vi "DiffDriveTrainSim_SetInputs.vi"(8 "BatteryVoltage":dbl=12.0, 9 "Right_Volts":dbl=1.0, 10 "Left_Volts":dbl=1.0, 11 "in DiffDriveTrainSim":T1 {"m_Motor"."Jr_KgM2" format="%13.5p"; "m_Motor"."L_H" format="%13.5p"; "m_Motor"."Kt_NMPerAmp" format="%13.5p"; "m_Motor"."KvINV_RadPerSecPerVolt" format="%13.5p"; "m_Motor"."R_Ohms" format="%13.5p"; "m_Motor"."FreeSpeed_RadPerSec" format="%13.5p"; "m_Motor"."FreeCurrent_Amps" format="%13.5p"; "m_Motor"."StallCurrent_Amps" format="%13.5p"; "m_Motor"."StallTorque_NM" format="%13.5p"; "m_Motor"."nominalVoltage_Volts" format="%13.5p"}) -> (0 "Size Coerced":bool, 3 "out DiffDriveTrainSim":T1 {"m_Motor"."Jr_KgM2" format="%13.5p"; "m_Motor"."L_H" format="%13.5p"; "m_Motor"."Kt_NMPerAmp" format="%13.5p"; "m_Motor"."KvINV_RadPerSecPerVolt" format="%13.5p"; "m_Motor"."R_Ohms" format="%13.5p"; "m_Motor"."FreeSpeed_RadPerSec" format="%13.5p"; "m_Motor"."FreeCurrent_Amps" format="%13.5p"; "m_Motor"."StallCurrent_Amps" format="%13.5p"; "m_Motor"."StallTorque_NM" format="%13.5p"; "m_Motor"."nominalVoltage_Volts" format="%13.5p"})   [LabVIEW 2019, in "Trajectory_Library.lvlib"]
doc: "Sets the applied voltage to the drivetrain. Note that positive voltage must make that side of the drivetrain travel forward (+X).\n \nInputs:\n - DiffDriveTraimSim -- Data cluster\n - leftVoltageVolts -- The left voltage.\n - rightVoltageVolts -- The right voltage.\n - BatteryVoltage -- Current battery voltage (volts) (Default = 12 volts)\n\nOutputs:\n - OutDiffDriveTraimSim -- Updated data cluster.\n - SizeCoerced -- If TRUE, an error occured. Execution may continue."
uses:
  Trajectory_Library.lvlib
  TypeDef/LINEAR_SYSTEM.ctl
  <vilib>/Analysis/Matrix/Datatypes/RealMatrix.ctl
  <vilib>/Analysis/Matrix/NI_Matrix.lvlib
  TypeDef/DCMOTOR.CTL
  TypeDef/DIFF_DRIVE_TRAIN_SIM.ctl
panel:
  # "<States, 1>"
  # "<Outputs, 1>"
  # "<Inputs, 1>"
  # "<Outputs, 1>"
  # "<States,States>"
  # "<States,Inputs>"
  # "<Outputs,States>"
  # "<Outputs,Inputs>"
  # "<States, 1>"
  # "<Outputs, 1>"
  # "<Inputs, 1>"
  # "<Outputs, 1>"
  # "<States,States>"
  # "<States,Inputs>"
  # "<Outputs,States>"
  # "<Outputs,Inputs>"
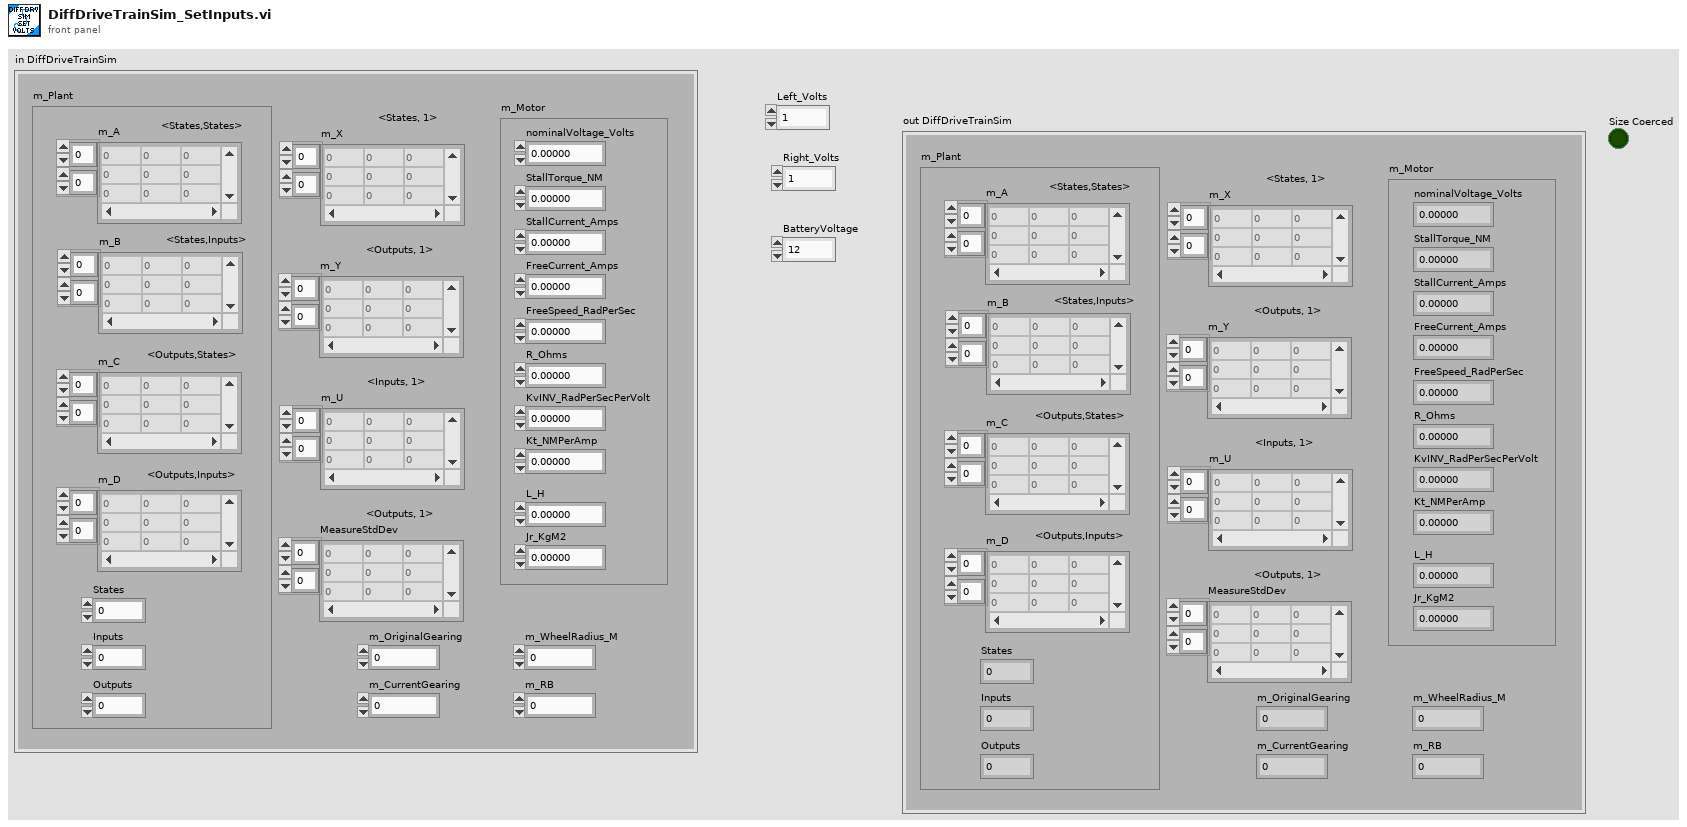
[diagram p1: front panel]
types:
  T1 = typedef "Trajectory_Library.lvlib/DIFF_DRIVE_TRAIN_SIM.ctl" = cluster{"m_Plant":T2, "m_X":T3, "m_Y":T3, "m_U":T3, "MeasureStdDev":T3, "m_Motor":T4, "m_OriginalGearing":dbl, "m_CurrentGearing":dbl, "m_WheelRadius_M":dbl, "m_RB":dbl}
  T2 = typedef "Trajectory_Library.lvlib/LINEAR_SYSTEM.ctl" = cluster{"m_A":T3, "m_B":T3, "m_C":T3, "m_D":T3, "States":i32, "Inputs":i32, "Outputs":i32}
  T3 = typedef "NI_Matrix.lvlib/RealMatrix.ctl" = dbl[][]
  T4 = typedef "Trajectory_Library.lvlib/DCMOTOR.CTL" = cluster{"nominalVoltage_Volts":dbl, "StallTorque_NM":dbl, "StallCurrent_Amps":dbl, "FreeCurrent_Amps":dbl, "FreeSpeed_RadPerSec":dbl, "R_Ohms":dbl, "KvINV_RadPerSecPerVolt":dbl, "Kt_NMPerAmp":dbl, "L_H":dbl, "Jr_KgM2":dbl}
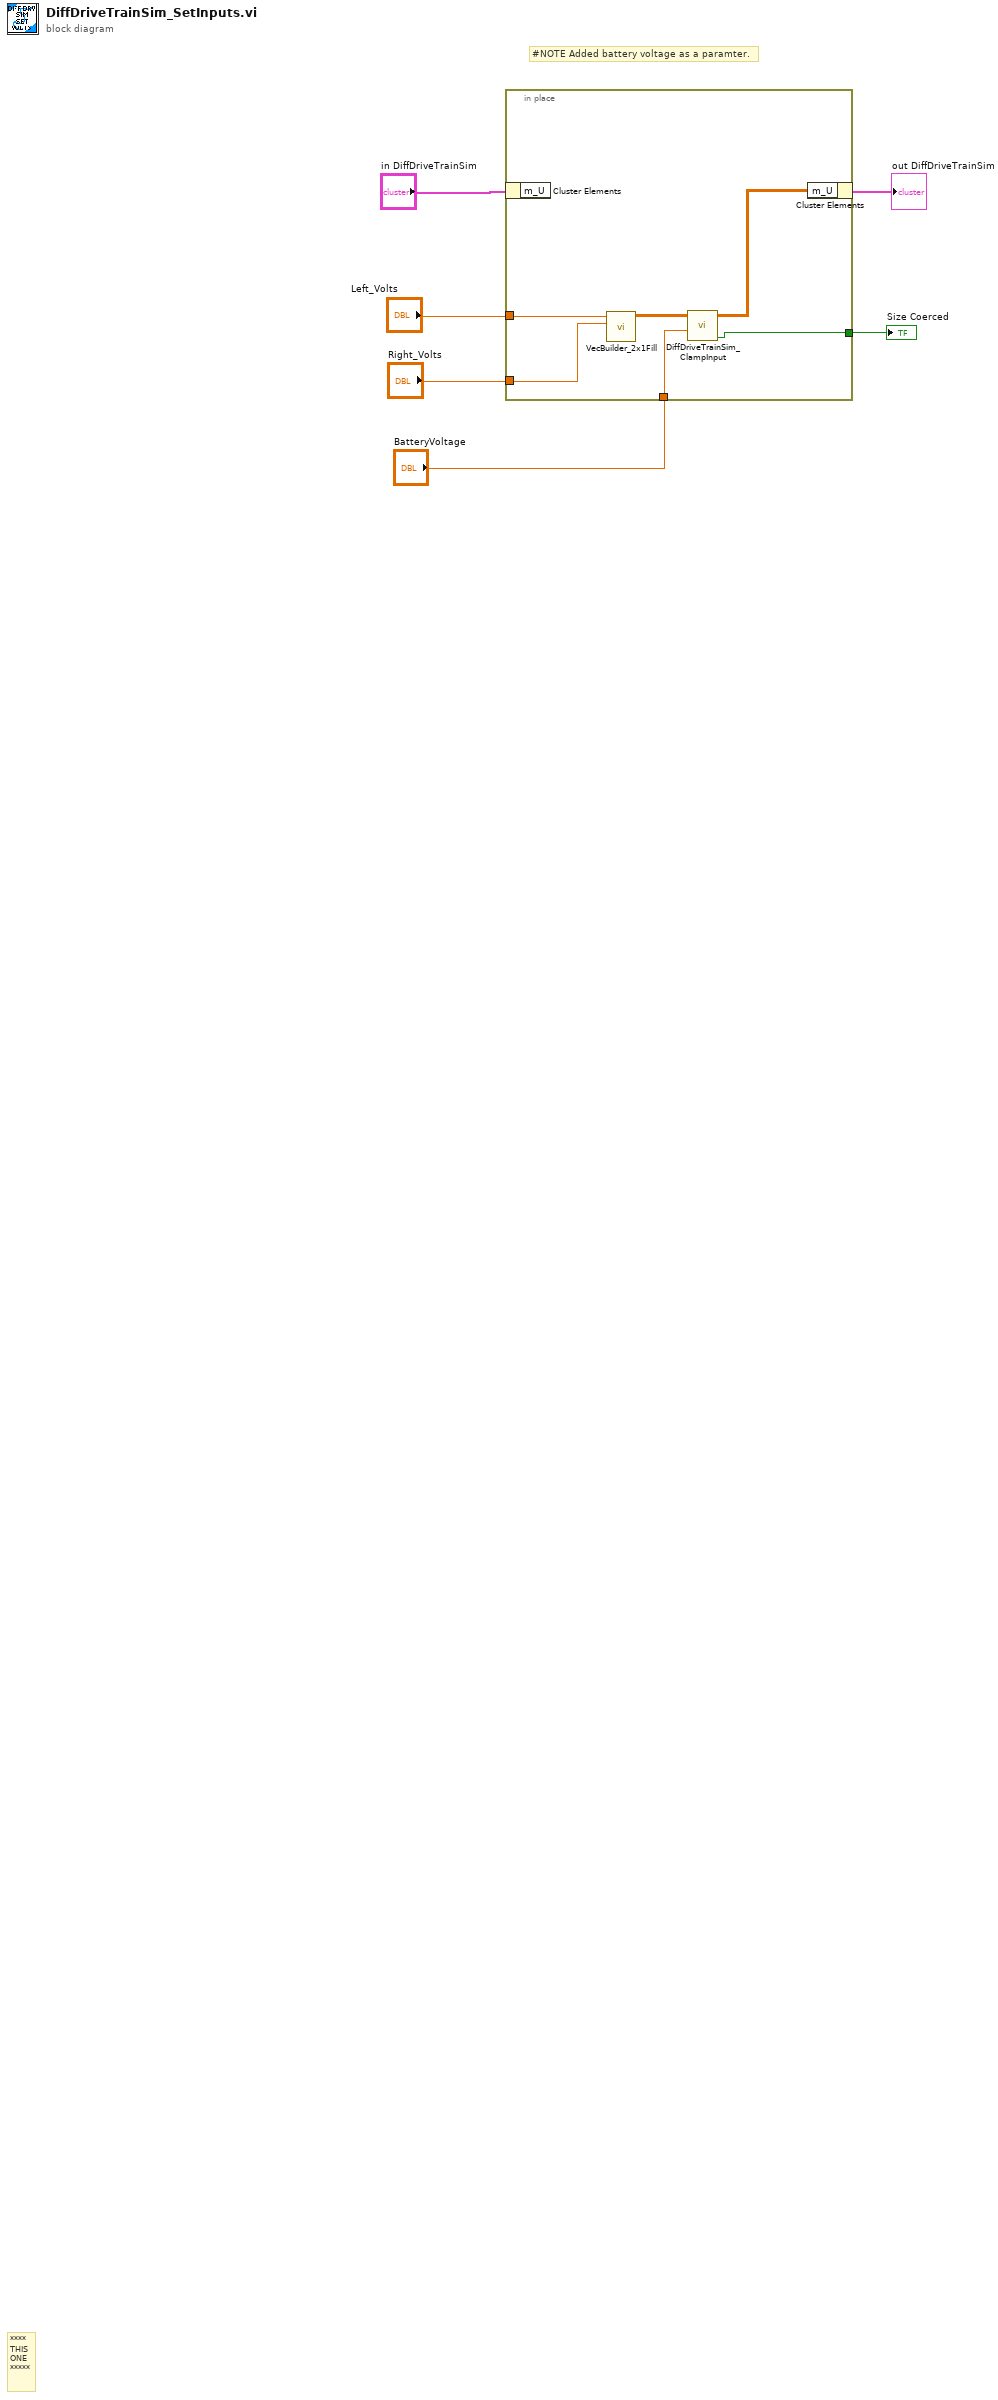
[diagram p0: block diagram]
diagram:
  # "#NOTE Added battery voltage as a paramter."
  # "****\nTHIS\nONE\n*****"
  n1 = in-place {
    in-place-border: "Left_Volts" -> [w12]
    in-place-border: "Right_Volts" -> [w11]
    in-place-border: "BatteryVoltage" -> [w8]
    in-place-border: [w7] -> w1
    n2 = in-place-cluster #1("in DiffDriveTrainSim") -> ()  [unwired: 1 out]
    n3 = call "VecBuilder_2x1Fill.vi"("R1"=w11, "R0"=w12) -> ("output matrix"=w10:T3)  [unwired: 9 in]
    n4 = call "DiffDriveTrainSim_ClampInput.vi"("BatteryVoltage"=w8, "U"=w10) -> ("Size Coerced"=w7:bool, "Normalized U"=w9:T3)  [unwired: 8 in]
    n5 = in-place-cluster #1("m_U"=w9) -> (→"out DiffDriveTrainSim":T1)
  }
  "Size Coerced" <- w1
